vi "rad_Load Config.vi"(8 "error in (no error":errorcluster, 11 "State in":T1 {"Targets Information"."Primary NIC"."IP Address Request Mode" items=["Static"=1, "DHCP/Link-Local"=2, "Link-Local Only"=4, "DHCP Only"=8]}) -> (0 "error out":errorcluster, 3 "State out":T1 {"Targets Information"."Primary NIC"."IP Address Request Mode" items=["Static"=1, "DHCP/Link-Local"=2, "Link-Local Only"=4, "DHCP Only"=8]})   [LabVIEW 2020]
uses:
  <vilib>/Utility/config.llb/NI_LVConfig.lvlib
  <vilib>/Utility/config.llb/Read Key (String).vi
  <vilib>/Utility/config.llb/Read Key (U32).vi
  <vilib>/Utility/config.llb/Read Key (Path).vi
  <vilib>/Utility/config.llb/Read Key (Boolean).vi
  <vilib>/Utility/config.llb/Read Key (I32).vi
  TypeDefs/rad_State Data.ctl
  Targets/TypeDefs/rad_Targets Settings.ctl
  support/SubVIs/Target Information.ctl
  Targets/TypeDefs/rad_Target Network Settings.ctl
  support/Controls/Discovery Settings.ctl
  support/Controls/Important Paths.ctl
  support/Controls/Discovery Method Enum.ctl
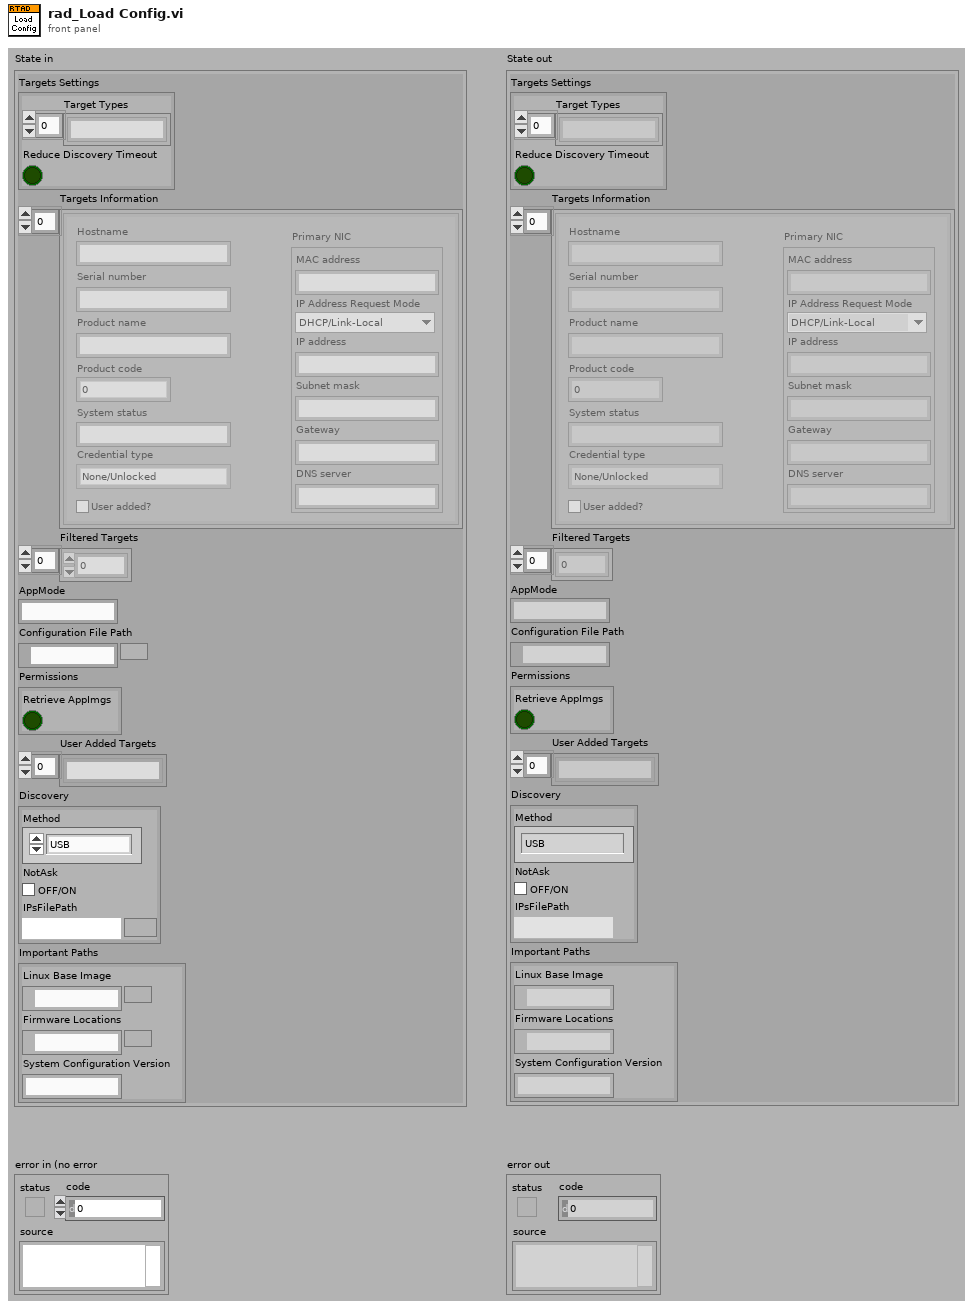
[diagram p1: front panel]
types:
  T1 = typedef "rad_State Data.ctl" = cluster{"Targets Settings":T2, "Targets Information":T3[], "Filtered Targets":i32[], "AppMode":string, "Configuration File Path":path, "Permissions":cluster{"Retrieve AppImgs":bool}, "User Added Targets":string[], "Discovery":T5, "Important Paths":T7}
  T2 = typedef "rad_Targets Settings.ctl" = cluster{"Target Types":string[], "Reduce Discovery Timeout":bool}
  T3 = typedef "Target Information.ctl" = cluster{"Hostname":string, "Serial number":string, "Product name":string, "Product code":i32, "System status":string, "Credential type":enum16{"None/Unlocked", "FTP Password", "NIAuth Credentials"}, "User added?":bool, "Primary NIC":T4}
  T4 = typedef "rad_Target Network Settings.ctl" = cluster{"MAC address":string, "IP Address Request Mode":i32, "IP address":string, "Subnet mask":string, "Gateway":string, "DNS server":string}
  T5 = typedef "Discovery Settings.ctl" = cluster{"Method":T6, "NotAsk":bool, "IPsFilePath":path}
  T6 = typedef "Discovery Method Enum.ctl" = enum32{"USB", "IPsFile", "AutoAll", "NotDiscover"}
  T7 = typedef "Important Paths.ctl" = cluster{"Linux Base Image":path, "Firmware Locations":path, "System Configuration Version":string}
  T8 = typedef "NI_LVConfig.lvlib/Config Data RefNum.ctl" = refnum<k1>
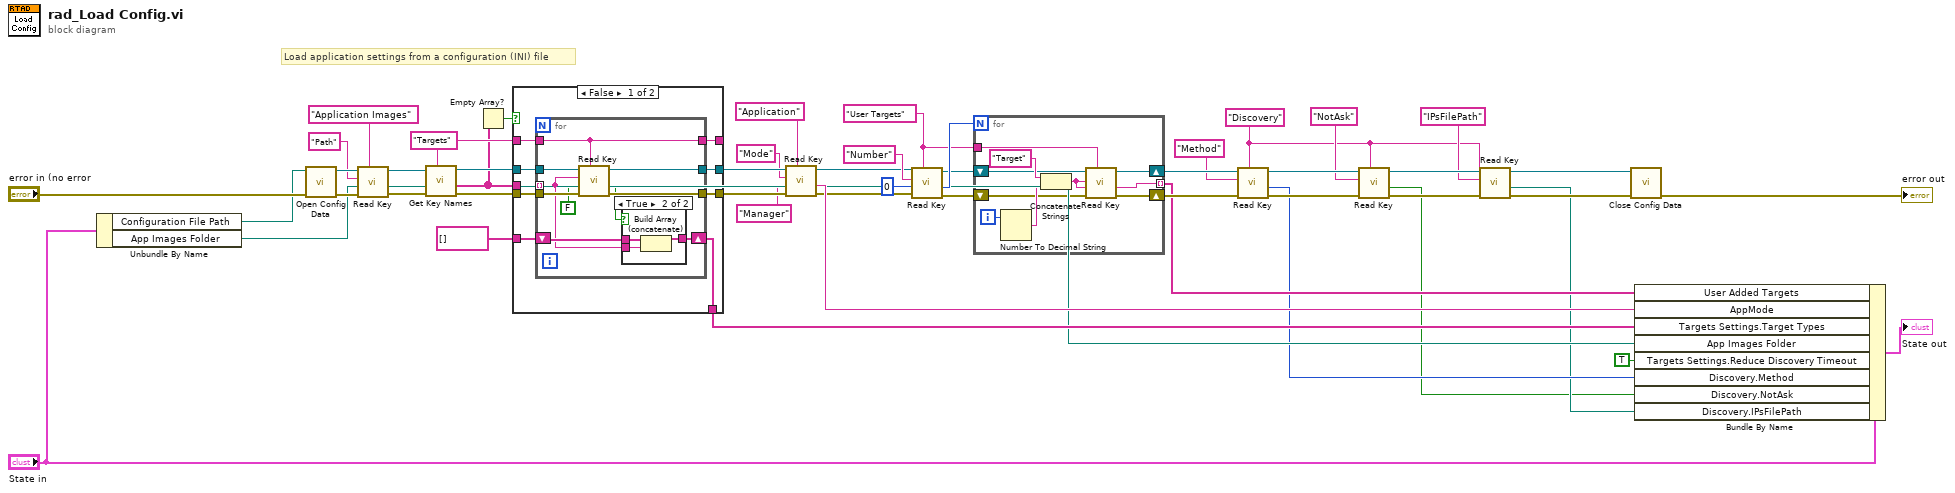
[diagram p0: block diagram]
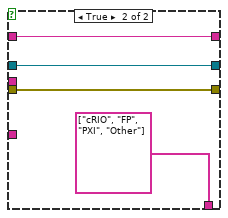
[diagram p3: hidden frame]
diagram:
  w1 = "Discovery" ("section")
  w25 = "User Targets" ("section")
  w44 = "Targets" ("section")
  # "Load application settings from a configuration (INI) file"
  n1 = Unbundle By Name("State in") -> ("Configuration File Path"=w16:path, "App Images Folder"=w30:path)
  n2 = call <vilib>:"Open Config Data.vi"("error in (no error)"="error in (no error", "configuration file path"=w16) -> ("error out"=w51:errorcluster, "refnum"=w50:T8)  [unwired: 7 in, 1 out]
  n3 = call-poly <vilib>:"Read Key.vi"("section"="Application Images", "error in (no error)"=w51, "default value"=w30, "key"="Path", "refnum"=w50) -> ("error out"=w46:errorcluster, "value"=w20:path, "refnum out"=w47:T8)  [unwired: 4 out]
  n4 = call <vilib>:"Get Key Names.vi"("section"=w44, "error in (no error)"=w46, "refnum"=w47) -> ("error out"=w45:errorcluster, "key names"=w40:string[], "refnum out"=w41:T8)  [unwired: 6 out]
  n5 = Empty Array?(array=w40) -> (empty?=w39:bool)
  n6 = case shown="False" w39 {
    tunnel: w45 -> [w60 w76]
    tunnel: w40 -> [w59 _]
    tunnel: w44 -> [w58 w78]
    tunnel: w41 -> [w57 w77]
    tunnel: [w54 w78] -> _
    tunnel: [w56 w77] -> w34
    tunnel: [w55 w76] -> w33
    tunnel: string[] [] ("Targets") -> [w53 _]
    tunnel: [w52 string[] ["cRIO", "FP", "PXI", "Other"] ("Targets")] -> w36
    frame False {
      n7 = for {
        tunnel: w60 -> [w70]
        tunnel: w57 -> [w68]
        tunnel: w59 -> [w61] mode=indexing
        tunnel: w58 -> [w69]
        tunnel: [w69] -> w54
        tunnel: [w67] -> w55
        tunnel: [w66] -> w56
        shift-right: [w62] -> w52
        shift-left: w53 -> [w63]
        n8 = call-poly <vilib>:"Read Key.vi"("section"=w69, "error in (no error)"=w70, "default value"=FALSE, "key"=w61, "refnum"=w68) -> ("error out"=w67:errorcluster, "value"=w64:bool, "refnum out"=w66:T8)  [unwired: 4 out]
        n9 = case shown="True" w64 {
          tunnel: w63 -> [w71 w74]
          tunnel: [w71 w73] -> w62
          tunnel: w61 -> [_ w72]
          frame False {
          }
          frame True {
            n10 = Build Array (concatenate)(w74, w72) -> (w73:string[])
          }
        }
      }
    }
    frame True {
    }
  }
  n11 = call-poly <vilib>:"Read Key.vi"("section"="Application", "error in (no error)"=w33, "default value"="Manager", "key"="Mode", "refnum"=w34) -> ("error out"=w18:errorcluster, "value"=w31:string, "refnum out"=w17:T8)  [unwired: 1 in, 3 out]
  n12 = call-poly <vilib>:"Read Key.vi"("section"=w25, "error in (no error)"=w18, "default value"=0 ("size(s)"), "key"="Number", "refnum"=w17) -> ("error out"=w24:errorcluster, "value"=w27:i32, "refnum out"=w26:T8)  [unwired: 4 out]
  n13 = for {
    N: w27 -> [_]
    tunnel: w25 -> [w82]
    shift-right: [w85] -> w23
    shift-left: w24 -> [w84]
    tunnel: [w79] -> w22 mode=indexing
    shift-right: [w80] -> w13
    shift-left: w26 -> [w81]
    i -> [w87]
    n14 = Number To Decimal String(number=w87) -> (decimal integer string=w88:string)  [unwired: 1 in]
    n15 = Concatenate Strings("Target" ("key"), w88) -> (w83:string)
    n16 = call-poly <vilib>:"Read Key.vi"("section"=w82, "error in (no error)"=w84, "default value"=w83, "key"=w83, "refnum"=w81) -> ("error out"=w85:errorcluster, "value"=w79:string, "refnum out"=w80:T8)  [unwired: 1 in, 3 out]
  }
  n17 = call-poly <vilib>:"Read Key.vi"("section"=w1, "error in (no error)"=w23, "key"="Method", "refnum"=w13) -> ("error out"=w14:errorcluster, "value"=w12:u32, "refnum out"=w9:T8)  [unwired: 4 in, 1 out]
  n18 = call-poly <vilib>:"Read Key.vi"("section"=w1, "error in (no error)"=w14, "key"="NotAsk", "refnum"=w9) -> ("error out"=w10:errorcluster, "value"=w4:bool, "refnum out"=w7:T8)  [unwired: 4 in, 1 out]
  n19 = call-poly <vilib>:"Read Key.vi"("section"=w1, "error in (no error)"=w10, "key"="IPsFilePath", "refnum"=w7) -> ("error out"=w8:errorcluster, "value"=w5:path, "refnum out"=w6:T8)  [unwired: 4 in, 1 out]
  n20 = call <vilib>:"Close Config Data.vi"("error in (no error)"=w8, "refnum"=w6) -> ("error out"=→"error out":errorcluster)  [unwired: 1 in, 8 out]
  n21 = Bundle By Name(cluster="State in", "User Added Targets"=w22, "AppMode"=w31, "Targets Settings.Target Types"=w36, "App Images Folder"=w20, "Targets Settings.Reduce Discovery Timeout"=TRUE, "Discovery.Method"=w12, "Discovery.NotAsk"=w4, "Discovery.IPsFilePath"=w5) -> (→"State out":T1)
